vi "Generate Scalar Output Aliases (SubVI).vi"(1 "Aliases Seed":string[](array[string])=["BOOL", "FXP", "I8", "I16", "I32", "I64", "SGL", "U8", "U16", "U32", "U64"]) -> (0 "Scalar Output Aliases":string[](array[string]))   [LabVIEW 2019, in "Scalar Channels Testing.lvclass"]
uses:
  Scalar Channels Testing.lvclass
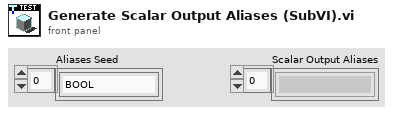
[diagram p1: front panel]
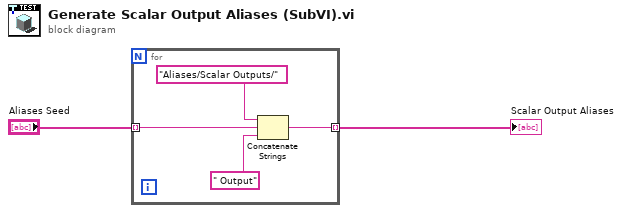
[diagram p0: block diagram]
diagram:
  n1 = for {
    tunnel: "Aliases Seed" -> [w4] mode=indexing
    tunnel: [w3] -> w2 mode=indexing
    n2 = Concatenate Strings("Aliases/Scalar Outputs/" ("string"), w4, " Output" ("string")) -> (w3:string)
  }
  "Scalar Output Aliases" <- w2
